vi "Read_340-file_v2.vi"() -> ()   [LabVIEW 2010]
uses:
  Instrument_Setup.vi
panel:
  out "Interpolated Termperature scalar":dbl
  out "Log Resistance":dbl
  in  "Resistance value":dbl
  in  "Nr of calibration data points":dbl
  out "Original Data":dbl[][](array[numeric]) caption="340 file to Array" format="%#.5g"
  out "xyz.340":string caption="340 file"
  in  "Pfad zu .340 file":path=path "D:/Thermometer/RuOxTL400_MK_Tail.340"
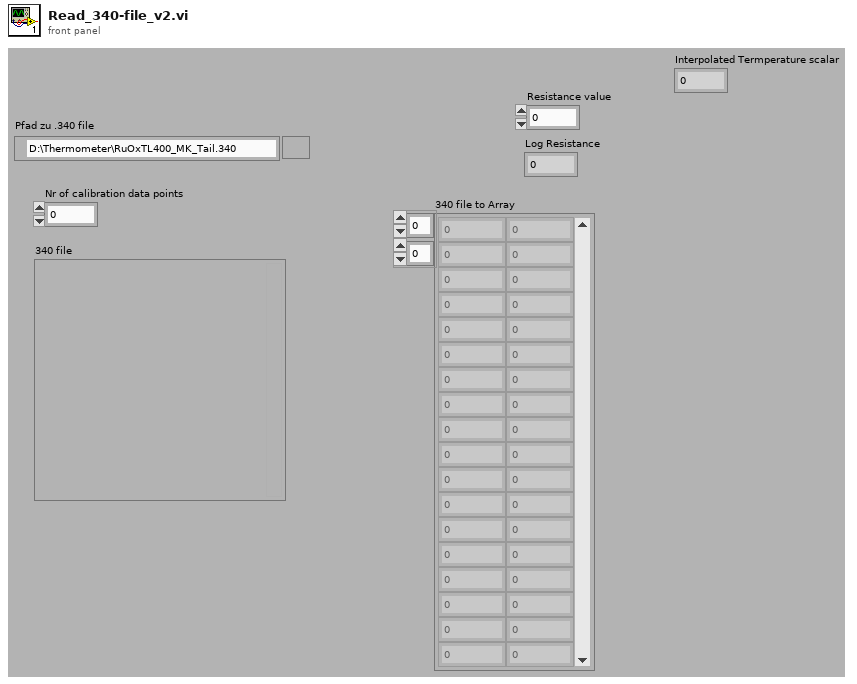
[diagram p1: front panel]
types:
  T1 = enum16{"open", "replace", "create", "open or create", "replace or create", "replace or create with confirmation"}
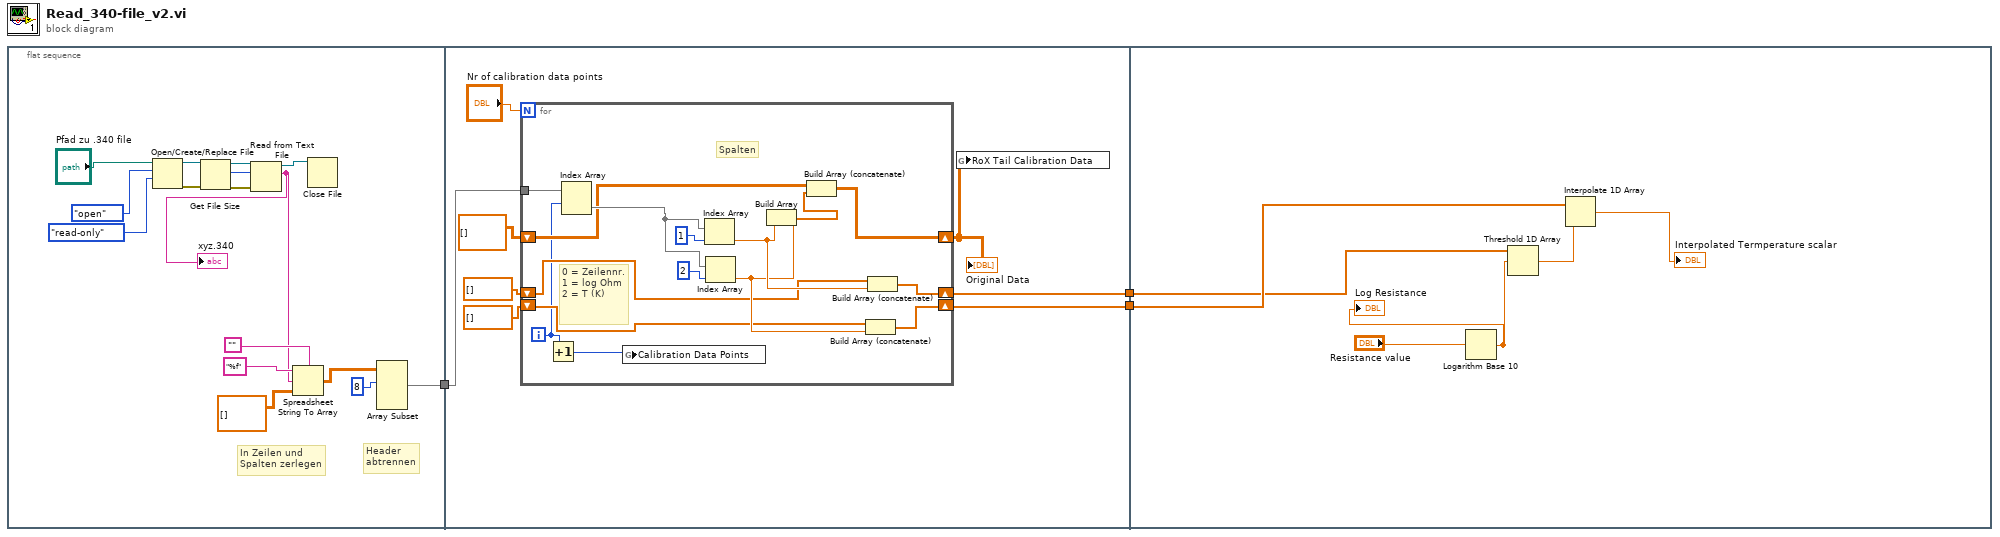
[diagram p0: block diagram]
diagram:
  n1 = flat-sequence {
    tunnel: [w6] -> w3
    tunnel: w3 -> [w27]
    tunnel: [w23] -> w2
    tunnel: [w22] -> w1
    tunnel: w2 -> [w44]
    tunnel: w1 -> [w45]
    frame #0 {
      # "In Zeilen und \nSpalten zerlegen"
      # "Header\nabtrennen"
      n2 = Open/Create/Replace File(file path (use dialog)="Pfad zu .340 file", operation (0:open)=T1."open", access (0:read/write)=enum16{"read/write", "read-only", "write-only"}."read-only") -> (refnum out=w14:refnum<file>, error out=w16:errorcluster)  [unwired: 3 in, 1 out]
      n3 = Get File Size(file=w14, error in=w16) -> (refnum out=w13:refnum<file>, size (in bytes)=w4:i64, 0:w15:errorcluster)
      n4 = Read from Text File(file (use dialog)=w13, count=w4, error in=w15) -> (refnum out=w12:refnum<file>, text=w9:string)  [unwired: 1 in, 2 out]
      "xyz.340" <- w9
      n5 = Spreadsheet String To Array(delimiter (Tab)="", format string="%f", spreadsheet string=w9, array type (2D Dbl)=dbl[][] []) -> (array=w5:dbl[][])
      n6 = Close File(refnum=w12) -> ()  [unwired: 1 in, 2 out]
      n7 = Array Subset(array=w5, index (row)=8) -> (w6:dbl[][])  [unwired: 3 in]
    }
    frame #1 {
      n8 = for {
        N: "Nr of calibration data points" -> [_]
        tunnel: w27 -> [w40]
        shift-right: [w37] -> w25
        shift-left: dbl[][] [] -> [w36]
        shift-right: [w35] -> w23
        shift-left: dbl[] [] -> [w31]
        shift-right: [w34] -> w22
        shift-left: dbl[] [] -> [w30]
        i -> [w29]
        # "0 = Zeilennr.\n1 = log Ohm\n2 = T (K)"
        # "Spalten"
        n9 = Increment(x=w29) -> (x+1=w28:i32)
        n10 = Index Array(array=w40, index (row)=w29) -> (element=w39:dbl[])  [unwired: 1 in]
        n11 = global write "Instrument_Setup.vi" "Calibration Data Points"(w28) -> ()
        n12 = Index Array(array=w39, index=1) -> (element=w33:dbl)
        n13 = Index Array(array=w39, index=2) -> (element=w32:dbl)
        n14 = Build Array(w33, w32) -> (w38:dbl[])
        n15 = Build Array (concatenate)(w36, w38) -> (w37:dbl[][])
        n16 = Build Array (concatenate)(w30, w32) -> (w34:dbl[])
        n17 = Build Array (concatenate)(w31, w33) -> (w35:dbl[])
      }
      "Original Data" <- w25
      n18 = global write "Instrument_Setup.vi" "RoX Tail Calibration Data"(w25) -> ()
    }
    frame #2 {
      n19 = Logarithm Base 10(1:"Resistance value") -> (0:w46:dbl)
      "Log Resistance" <- w46
      n20 = Threshold 1D Array(2:w46, 3:w44) -> (0:w47:dbl)  [unwired: 1 in]
      n21 = Interpolate 1D Array(1:w47, 2:w45) -> (0:→"Interpolated Termperature scalar":dbl)
    }
  }
